vi "MGCC_Commun_lowpassfilter.vi"(10 "Col":i32) -> ()   [LabVIEW 2016]
uses:
  <vilib>/Analysis/baseanly.llb/Mean (DBL).vi
  Global communication.vi
  Model Management/Global_MdlMgmt.vi
  <vilib>/Analysis/NI_AALBase.lvlib
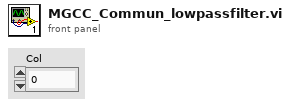
[diagram p1: front panel]
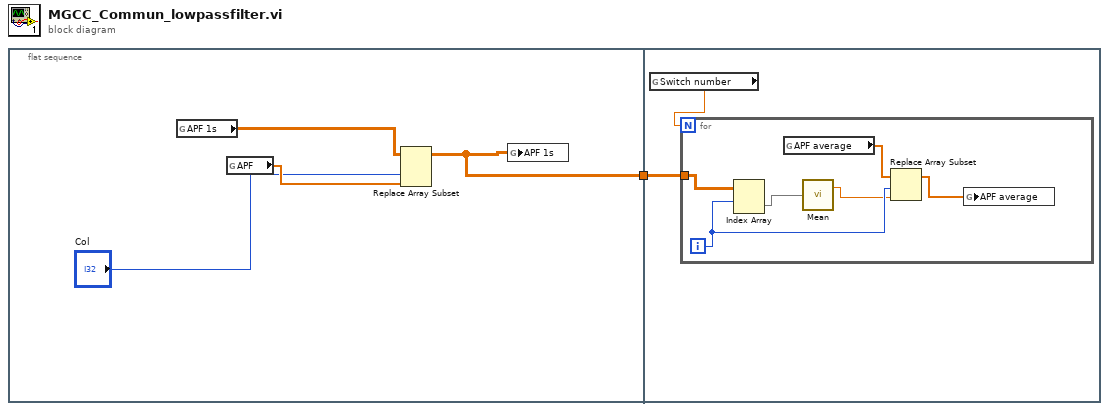
[diagram p0: block diagram]
diagram:
  n1 = flat-sequence {
    tunnel: [w2] -> w1
    tunnel: w1 -> [w7]
    frame #0 {
      n2 = global read "Global communication.vi" "APF 1s"() -> (w4:dbl[][])
      n3 = global read "Global communication.vi" "APF"() -> (w5:dbl[])
      n4 = Replace Array Subset(array=w4, new element=w5, index (col)="Col") -> (w2:dbl[][])  [unwired: 1 in]
      n5 = global write "Global communication.vi" "APF 1s"(w2) -> ()
    }
    frame #1 {
      n6 = global read "Global_MdlMgmt.vi" "Switch number"() -> (w6:dbl)
      n7 = for {
        N: w6 -> [_]
        tunnel: w7 -> [w13]
        i -> [w10]
        n8 = Index Array(array=w13, index (row)=w10) -> (element=w12:dbl[])  [unwired: 1 in]
        n9 = global read "Global communication.vi" "APF average"() -> (w11:dbl[])
        n10 = call-poly <vilib>:"Mean.vi"("X"=w12) -> ("mean"=w9:dbl)  [unwired: 1 out]
        n11 = Replace Array Subset(array=w11, new element=w9, index=w10) -> (w8:dbl[])
        n12 = global write "Global communication.vi" "APF average"(w8) -> ()
      }
    }
  }
